vi "Teleop.vi"(10 "Match Info":T1={"Autonomous Elapsed Seconds"=0.0, "TeleOp Elapsed Seconds"=0.0, "Disabled Elapsed Seconds"=0.0, "Visited Autonomous"=FALSE, "Visited TeleOp"=FALSE, "Visited Disabled"=FALSE, "Autonomous Settings"={"Autonomous Style"=enum."Independent", "VI Refnum"=refnum}}, 11 "Call Context":T2) -> ()   [LabVIEW 2013]
doc: "This VI is called for each TeleOp packet received from the DS where the robot is not disabled. It is often used to read from the joysticks and update I/O or to update setpoints for timed control loops. It should complete and return within 20 milliseconds or it may miss DS packets."
uses:
  <vilib>/Rock Robotics/WPI/DriverStation/WPI_DriverStationDerivedRobotMode.ctl
  <vilib>/Rock Robotics/WPI/DriverStation/WPI_DriverStationMatch Info.ctl
  Robot Global Data.vi
  <vilib>/Rock Robotics/WPI/Joystick/WPI_JoystickGetSetRefNum.vi
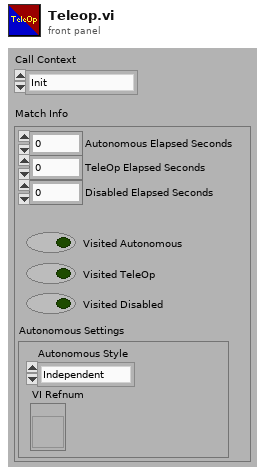
[diagram p1: front panel]
types:
  T1 = typedef "WPI_DriverStationMatch Info.ctl" = cluster{"Autonomous Elapsed Seconds":dbl, "TeleOp Elapsed Seconds":dbl, "Disabled Elapsed Seconds":dbl, "Visited Autonomous":bool, "Visited TeleOp":bool, "Visited Disabled":bool, "Autonomous Settings":cluster{"Autonomous Style":enum16{"Iterative", "Independent"}, "VI Refnum":refnum<vi>}}
  T2 = typedef "WPI_DriverStationDerivedRobotMode.ctl" = enum16{"Init", "Execute", "Stop"}
  T3 = typedef "WPI_JoystickDevRef.ctl" = cluster{"Device":T4}
  T4 = typedef "WPI_JoystickDeviceEnum.ctl" = enum16{"USB 1", "USB 2", "USB 3", "USB 4", "Kinect 1", "Kinect 2"}
  T5 = typedef "WPI_JoystickButtonState.ctl" = cluster{"Button 1":bool, "Button 2":bool, "Button 3":bool, "Button 4":bool, "Button 5":bool, "Button 6":bool, "Button 7":bool, "Button 8":bool, "Button 9":bool, "Button 10":bool, "Button 11":bool, "Button 12":bool}
  T6 = cluster{"axis 1 (x)":dbl, "axis 2 (y)":dbl, "axis 3 (throttle)":dbl, "axis 4":dbl, "axis 5":dbl, "axis 6":dbl}
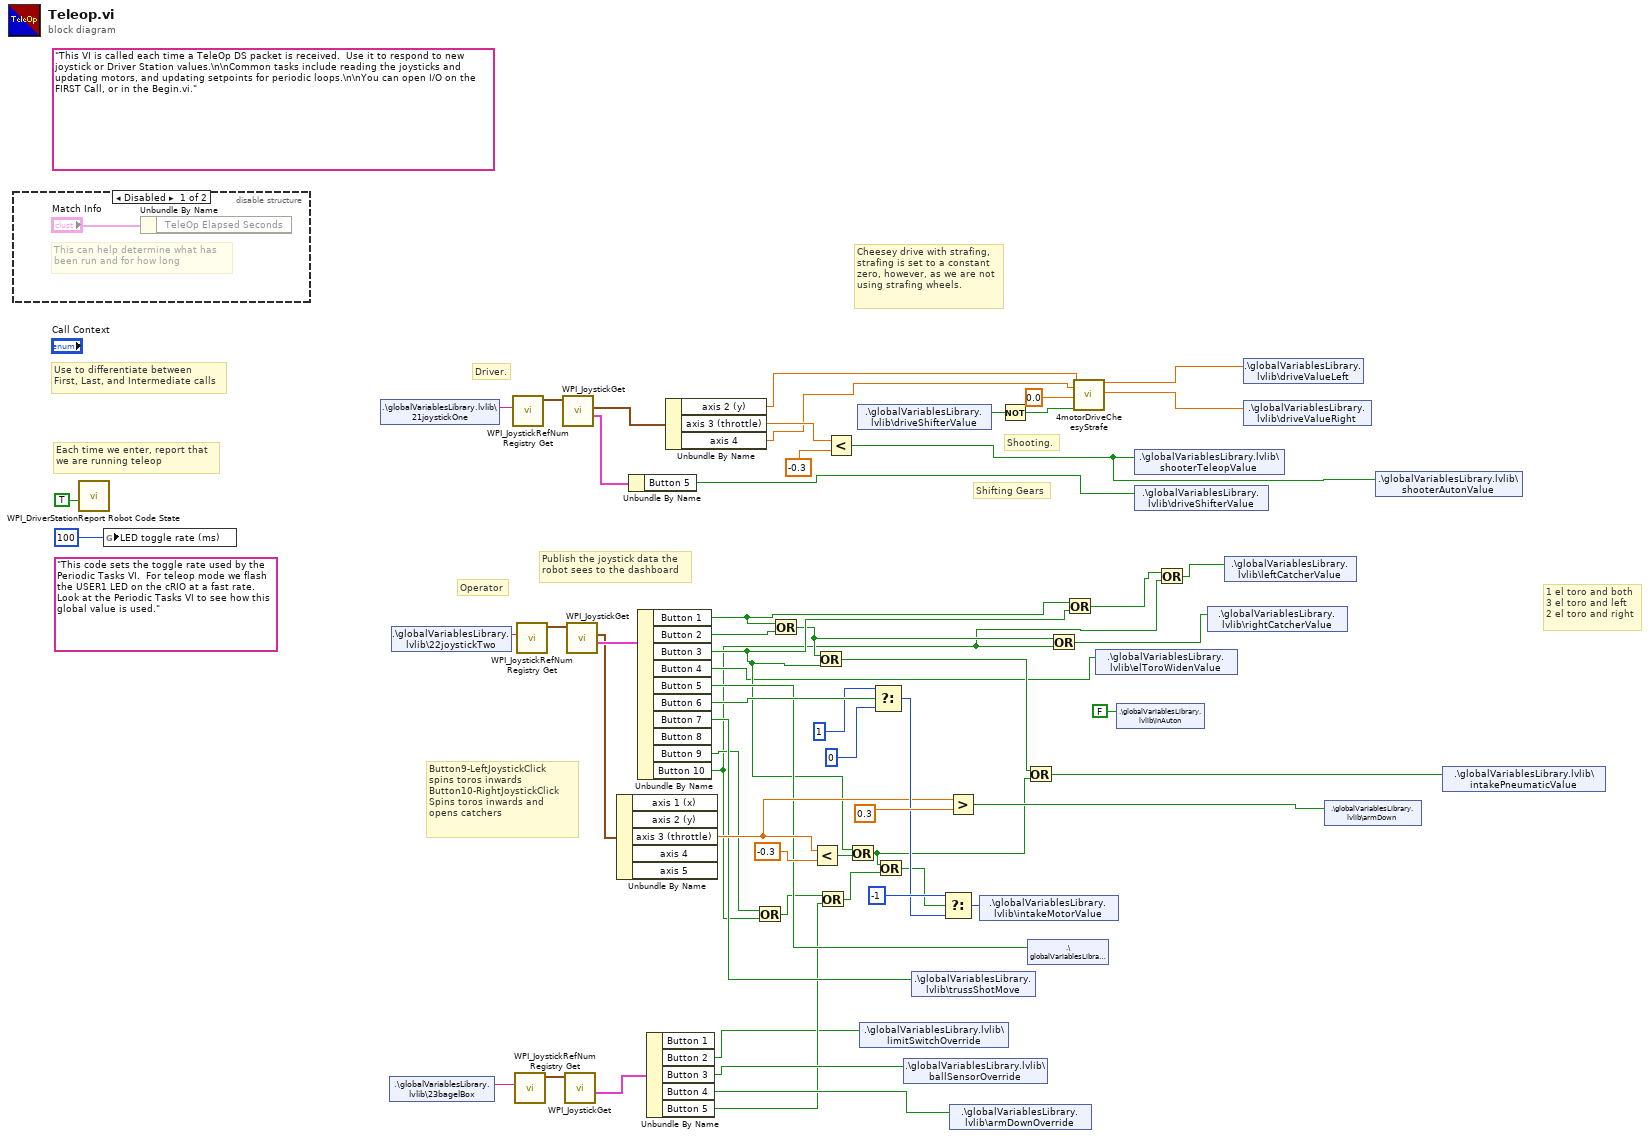
[diagram p0: block diagram]
diagram:
  (unwired) "This code sets the toggle rate used by the Periodic Tasks VI.  For teleop mode we flash the USER1 LED on the cRIO at a fast rate.  Look at the Periodic Tasks VI to see how this global value is used."
  (unwired) "This VI is called each time a TeleOp DS packet is received.  Use it to respond to new joystick or Driver Station values.\n\nCommon tasks include reading the joysticks and updating motors, and updating setpoints for periodic loops.\n\nYou can open I/O on the FIRST Call, or in the Begin.vi."
  # "Button9-LeftJoystickClick\nspins toros inwards\nButton10-RightJoystickClick\nSpins toros inwards and \nopens catchers"
  # "1 el toro and both\n3 el toro and left\n2 el toro and right"
  # "Shifting Gears"
  # "Driver."
  # "Operator"
  # "Shooting."
  # "Publish the joystick data the\nrobot sees to the dashboard"
  # "Cheesey drive with strafing, strafing is set to a constant zero, however, as we are not using strafing wheels."
  # "Each time we enter, report that\nwe are running teleop"
  # "Use to differentiate between\nFirst, Last, and Intermediate calls"
  n1 = disable-structure shown="Disabled" {
    frame Disabled {
      # "This can help determine what has\nbeen run and for how long"
      n2 = Unbundle By Name("Match Info") -> ()  [unwired: 1 out]
    }
    frame Enabled {
    }
  }
  n3 = call <vilib>:"WPI_DriverStationReport Robot Code State.vi"("TeleOp"=TRUE ("Autonomous")) -> ()  [unwired: 10 in, 1 out]
  n4 = global write "Robot Global Data.vi" "LED toggle rate (ms)"(u32 100 ("LED ms toggle rate")) -> ()
  n5 = shared-variable ".\\globalVariablesLibrary.lvlib\\21joystickOne"() -> (w52:string)  [unwired: 1 in, 1 out]
  n6 = shared-variable ".\\globalVariablesLibrary.lvlib\\23bagelBox"() -> (w18:string)  [unwired: 1 in, 1 out]
  n7 = shared-variable ".\\globalVariablesLibrary.lvlib\\22joystickTwo"() -> (w49:string)  [unwired: 1 in, 1 out]
  n8 = call <vilib>:"WPI_JoystickRefNum Registry Get.vi"("refnum name"=w52) -> ("JoystickDevRef"=w58:T3)  [unwired: 1 in, 9 out]
  n9 = call <vilib>:"WPI_JoystickRefNum Registry Get.vi"("refnum name"=w18) -> ("JoystickDevRef"=w17:T3)  [unwired: 1 in, 9 out]
  n10 = call <vilib>:"WPI_JoystickRefNum Registry Get.vi"("refnum name"=w49) -> ("JoystickDevRef"=w50:T3)  [unwired: 1 in, 9 out]
  n11 = call <vilib>:"WPI_JoystickGet.vi"("JoystickDevRef"=w58) -> ("Buttons"=w31:T5, "Axes"=w55:T6)  [unwired: 1 in, 4 out]
  n12 = call <vilib>:"WPI_JoystickGet.vi"("JoystickDevRef"=w17) -> ("Buttons"=w16:T5)  [unwired: 1 in, 5 out]
  n13 = call <vilib>:"WPI_JoystickGet.vi"("JoystickDevRef"=w50) -> ("Buttons"=w48:T5, "Axes"=w47:T6)  [unwired: 1 in, 4 out]
  n14 = Unbundle By Name(w47) -> ("axis 3 (throttle)"=w33:dbl)  [unwired: 4 out]
  n15 = Unbundle By Name(w31) -> ("Button 5"=w30:bool)
  n16 = Unbundle By Name(w48) -> ("Button 1"=w34:bool, "Button 2"=w37:bool, "Button 3"=w20:bool, "Button 4"=w19:bool, "Button 5"=w23:bool, "Button 6"=w43:bool, "Button 7"=w24:bool, "Button 9"=w9:bool, "Button 10"=w4:bool)  [unwired: 1 out]
  n17 = Unbundle By Name(w16) -> ("Button 2"=w1:bool, "Button 3"=w12:bool, "Button 4"=w13:bool, "Button 5"=w11:bool)  [unwired: 1 out]
  n18 = Unbundle By Name(w55) -> ("axis 2 (y)"=w27:dbl, "axis 3 (throttle)"=w32:dbl, "axis 4"=w26:dbl)
  n19 = Or(x=w9, y=w4) -> (x .or. y?=w8:bool)
  n20 = Or(x=w34, y=w37) -> (x .or. y?=w7:bool)
  n21 = Less?(x=w33, y=-0.3) -> (x < y?=w35:bool)
  n22 = Or(x=w7, y=w20) -> (x .or. y?=w36:bool)
  n23 = Or(x=w8, y=w11) -> (x .or. y?=w10:bool)
  n24 = Less?(x=w32, y=-0.3) -> (x < y?=w21:bool)
  n25 = Or(x=w20, y=w35) -> (x .or. y?=w15:bool)
  n26 = shared-variable ".\\globalVariablesLibrary.lvlib\\driveShifterValue"() -> (w29:bool)  [unwired: 1 in, 1 out]
  n27 = shared-variable ".\\globalVariablesLibrary.lvlib\\limitSwitchOverride"(w1) -> ()  [unwired: 1 in, 1 out]
  n28 = Select(t=1, s=w43, f=0) -> (s? t:f=w38:i32)
  n29 = Or(x=w15, y=w10) -> (x .or. y?=w14:bool)
  n30 = shared-variable ".\\globalVariablesLibrary.lvlib\\ballSensorOverride"(w12) -> ()  [unwired: 1 in, 1 out]
  n31 = shared-variable ".\\globalVariablesLibrary.lvlib\\trussShotMove"(w24) -> ()  [unwired: 1 in, 1 out]
  n32 = Select(t=-1, s=w14, f=w38) -> (s? t:f=w45:i32)
  n33 = Greater?(x=w33, y=0.3) -> (0:w25:bool)
  n34 = shared-variable ".\\globalVariablesLibrary.lvlib\\armDownOverride"(w13) -> ()  [unwired: 1 in, 1 out]
  n35 = shared-variable ".\\globalVariablesLibrary.lvlib\\intakeMotorValue"(w45) -> ()  [unwired: 1 in, 1 out]
  n36 = Not(x=w29) -> (.not. x?=w28:bool)
  n37 = Or(x=w36, y=w15) -> (x .or. y?=w22:bool)
  n38 = shared-variable ".\\globalVariablesLibrary.lvlib\\armUp"(w23) -> ()  [unwired: 1 in, 1 out]
  n39 = Or(x=w7, y=w4) -> (x .or. y?=w6:bool)
  n40 = Or(x=w34, y=w20) -> (x .or. y?=w5:bool)
  n41 = call "4motorDriveCheesyStrafe.vi"("Throttle"=w27, "Steering"=w26, "Strafing"=0.0, "Gear"=w28) -> ("leftMotors"=w54:dbl, "rightMotors"=w53:dbl)  [unwired: 14 in]
  n42 = shared-variable ".\\globalVariablesLibrary.lvlib\\elToroWidenValue"(w19) -> ()  [unwired: 1 in, 1 out]
  n43 = shared-variable ".\\globalVariablesLibrary.lvlib\\inAuton"(FALSE ("inAuton")) -> ()  [unwired: 1 in, 1 out]
  n44 = shared-variable ".\\globalVariablesLibrary.lvlib\\shooterTeleopValue"(w21) -> ()  [unwired: 1 in, 1 out]
  n45 = shared-variable ".\\globalVariablesLibrary.lvlib\\driveShifterValue"(w30) -> ()  [unwired: 1 in, 1 out]
  n46 = Or(x=w5, y=w4) -> (x .or. y?=w3:bool)
  n47 = shared-variable ".\\globalVariablesLibrary.lvlib\\rightCatcherValue"(w6) -> ()  [unwired: 1 in, 1 out]
  n48 = shared-variable ".\\globalVariablesLibrary.lvlib\\leftCatcherValue"(w3) -> ()  [unwired: 1 in, 1 out]
  n49 = shared-variable ".\\globalVariablesLibrary.lvlib\\driveValueLeft"(w54) -> ()  [unwired: 1 in, 1 out]
  n50 = shared-variable ".\\globalVariablesLibrary.lvlib\\driveValueRight"(w53) -> ()  [unwired: 1 in, 1 out]
  n51 = shared-variable ".\\globalVariablesLibrary.lvlib\\armDown"(w25) -> ()  [unwired: 1 in, 1 out]
  n52 = shared-variable ".\\globalVariablesLibrary.lvlib\\shooterAutonValue"(w21) -> ()  [unwired: 1 in, 1 out]
  n53 = shared-variable ".\\globalVariablesLibrary.lvlib\\intakePneumaticValue"(w22) -> ()  [unwired: 1 in, 1 out]
